vi "Menu Build File Item.vi"() -> (3 "Menu File Item":refnum<data-value>)   [LabVIEW 2018, in "Main Panel.lvlib" / "Main Panel.lvclass"]
uses:
  Main Panel.lvclass
  <userlib>/_MGI/Menu Building/MenuItem/MGI_MenuItem.lvclass
  Menu item.ctl
  <userlib>/_MGI/Menu Building/MenuItem/MenuSeparatorItem/MGI_MenuSeparatorItem.lvclass
  C:/Program Files (x86)/National Instruments/LabVIEW 2018/user.lib/_MGI/Menu Building/MenuItem/MGI_MenuItem.lvclass
  <userlib>/_MGI/Menu Building/MenuItem/MenuItem.vi
  <userlib>/_MGI/Menu Building/MenuItem/MenuSeparatorItem/MenuSeparatorItem.vi
  <userlib>/_MGI/Menu Building/MenuItem/Write Sub-Menus.vi
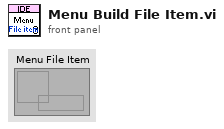
[diagram p1: front panel]
types:
  T1 = typedef "Main Panel.lvlib/Main Panel.lvclass/Menu Item.ctl" = enum16{"Invalid Item", "File", "Open File", "Save File", "Exit", "Settings", "Preferences", "Help", "Show Context Help"}
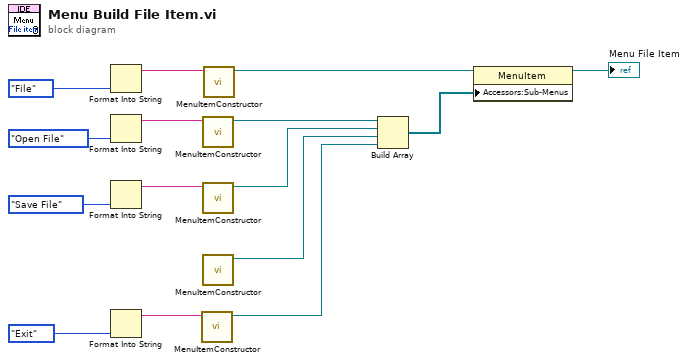
[diagram p0: block diagram]
diagram:
  n1 = Format Into String(Menu_Item."File" ("Menu item")) -> (resulting string=w1:string)  [unwired: 3 in, 1 out]
  n2 = Format Into String(Menu_Item."Open File" ("Menu item")) -> (resulting string=w10:string)  [unwired: 3 in, 1 out]
  n3 = Format Into String(Menu_Item."Save File" ("Menu item")) -> (resulting string=w8:string)  [unwired: 3 in, 1 out]
  n4 = Format Into String(Menu_Item."Exit" ("Menu item")) -> (resulting string=w3:string)  [unwired: 3 in, 1 out]
  n5 = call-poly <userlib>:"MenuItemConstructor.vi"("Text"=w3) -> ("MenuItem"=w4:refnum<data-value>)  [unwired: 9 in, 1 out]
  n6 = call-poly <userlib>:"MenuItemConstructor.vi"("Text"=w10) -> ("MenuItem"=w14:refnum<data-value>)  [unwired: 9 in, 1 out]
  n7 = call-poly <userlib>:"MenuItemConstructor.vi"("Text"=w8) -> ("MenuItem"=w6:refnum<data-value>)  [unwired: 9 in, 1 out]
  n8 = call-poly <userlib>:"MenuItemConstructor.vi"() -> ("MenuSeparatorItem"=w13:refnum<data-value>)  [unwired: 10 in, 1 out]
  n9 = call-poly <userlib>:"MenuItemConstructor.vi"("Text"=w1) -> ("MenuItem"=w15:refnum<data-value>)  [unwired: 9 in, 1 out]
  n10 = Build Array(w14, w6, w13, w4) -> (w12:refnum<data-value>[])
  n11 = property class="MenuItem"(reference=w15, "Accessors:Sub-Menus"=w12) -> (reference out=→"Menu File Item":refnum<data-value>)  [unwired: 1 in, 1 out]
